vi "Stop Core.vi"(10 "final error code":i32, 11 "Vehicle Position Simulation in":refnum<class "Vehicle Position Simulation.lvclass">) -> (3 "Vehicle Position Simulation out":refnum<class "Vehicle Position Simulation.lvclass">)   [LabVIEW 2019, in "Vehicle Position Simulation.lvlib" / "Vehicle Position Simulation.lvclass"]
doc: "(<B>Filename</B>: Actor Framework.lvlib:Actor.lvclass:Stop Core.vi)\n\nDefines what the actor does before it stops. Use the <B>final error code</B> input to determine whether the actor shut down in response to an error.\n\nBy default, this method passes the Stop message along to all auto-stop nested actors. A descendant class may override this method to define additional behavior, such as shutting down any processes the actor initiated in its override of the Actor Core method."
uses:
  Vehicle Position Simulation.lvclass
  Vehicle Position Simulation.lvclass/Vehicle Position Simulation.ctl
  Abstract Vehicle Position Interface/Abstract Vehicle Position Interface/Vehicle Position Interface.lvclass
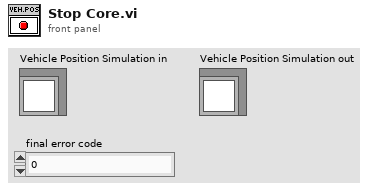
[diagram p1: front panel]
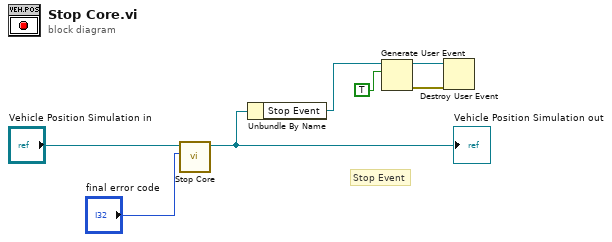
[diagram p0: block diagram]
diagram:
  # "Stop Event"
  n1 = call-parent "Stop Core.vi"("final error code"="final error code", "Actor in"="Vehicle Position Simulation in") -> ("Actor out"=w1:refnum<class "Vehicle Position Simulation.lvclass">)  [unwired: 9 in]
  "Vehicle Position Simulation out" <- w1
  n2 = Unbundle By Name(w1) -> ("Stop Event"=w3:refnum<user-event>)
  n3 = Generate User Event(user event=w3, event data cluster=TRUE ("event data")) -> (user event out=w5:refnum<user-event>, error out=w4:errorcluster)  [unwired: 2 in]
  n4 = Destroy User Event(user event=w5, error in=w4) -> ()  [unwired: 1 out]
